vi "Init.vi"(8 "error in (no error)":errorcluster, 9 "Team":refnum<class "Team.lvclass">, 10 "Remove Team":refnum<user-event>, 11 "Start Position":refnum<user-event>) -> (0 "error out":errorcluster, 3 "Team Config Panel out":refnum<class "Team Config Panel.lvclass">)   [LabVIEW 2020, in "SB App.lvlib" / "Team Config Panel.lvclass"]
uses:
  Team Config Panel.lvclass
  SquareBattle/Team/Team.lvclass
  SquareBattle/Team ID.ctl
  Start Position Data.ctl
  SquareBattle/Position.ctl
  Team Config Panel.lvclass/Team Config Panel.ctl
  SquareBattle/SquareBattle.lvlib
  SB App.lvlib
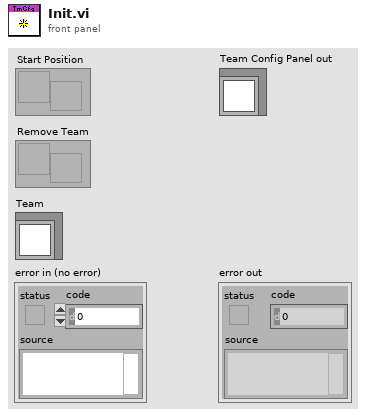
[diagram p1: front panel]
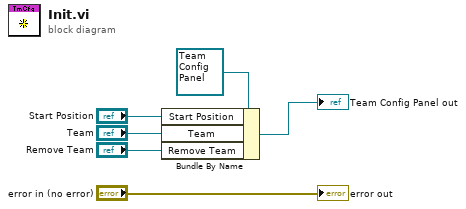
[diagram p0: block diagram]
diagram:
  n1 = Bundle By Name(cluster=refnum<class "Team Config Panel.lvclass"> refnum ("Team Config Panel in"), "Start Position"="Start Position", "Team"="Team", "Remove Team"="Remove Team") -> (→"Team Config Panel out":refnum<class "Team Config Panel.lvclass">)
  "error out" <- "error in (no error)"
